vi "Acquire and Time.vi"(7 "samples per block":i64=-1, 8 "error in (no error)":errorcluster, 11 "RFSA Reference In":refnum<k15>) -> (0 "error out":errorcluster, 1 "bytes":i32, 2 "data":waveform(cdb), 3 "RFSA Reference Out":refnum<k15>, 5 "DAQ B/sec":dbl caption="ACQUISITION RATE")   [LabVIEW 2021]
uses:
  <instrlib>/niRFSA/niRFSA.llb/niRFSA Fetch IQ (Complex WDT 1Rec 1Chan).vi
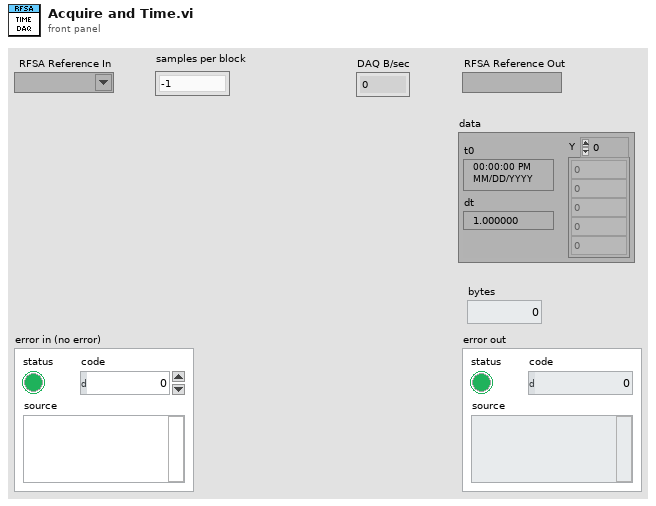
[diagram p1: front panel]
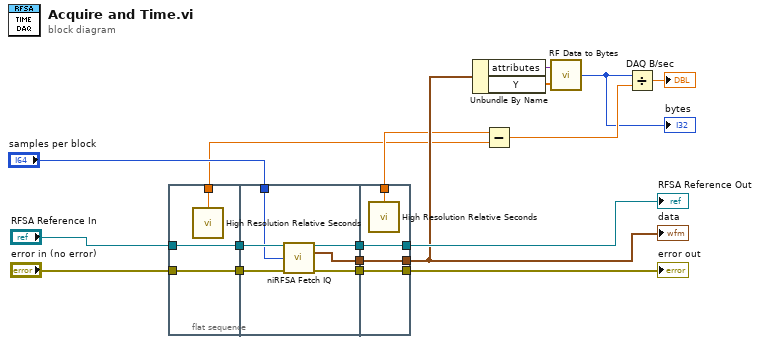
[diagram p0: block diagram]
diagram:
  n1 = flat-sequence {
    tunnel: [w19] -> w3
    tunnel: [w21] -> w18
    tunnel: "error in (no error)" -> [w21]
    tunnel: "RFSA Reference In" -> [w20]
    tunnel: [w20] -> w17
    tunnel: w18 -> [w27]
    tunnel: [w26] -> w16
    tunnel: [w25] -> w15
    tunnel: [w24] -> w14
    tunnel: w17 -> [w23]
    tunnel: "samples per block" -> [w22]
    tunnel: [w28] -> w4
    tunnel: w16 -> [w31]
    tunnel: [w31] -> w11
    tunnel: [w30] -> w5
    tunnel: w15 -> [w30]
    tunnel: w14 -> [w29]
    tunnel: [w29] -> w12
    frame #0 {
      n2 = call <vilib>:"High Resolution Relative Seconds.vi"() -> ("relative seconds"=w19:dbl)
    }
    frame #1 {
      n3 = call-poly <instrlib>:"niRFSA Fetch IQ.vi"("instrument handle"=w23, "samples to read (-1)"=w22, "error in"=w27) -> ("instrument handle out"=w24:refnum<k15>, "data"=w25:waveform(cdb), "error out"=w26:errorcluster)  [unwired: 10 in]
    }
    frame #2 {
      n4 = call <vilib>:"High Resolution Relative Seconds.vi"() -> ("relative seconds"=w28:dbl)
    }
  }
  n5 = Unbundle By Name(w5) -> ("attributes"=w7:variant, "Y"=w8:cdb[])
  n6 = Subtract(x=w4, y=w3) -> (x-y=w2:dbl)
  n7 = call "RF Data to Bytes.vi"("Y"=w8, "attributes"=w7) -> ("Bytes"=w1:i32)
  "bytes" <- w1
  n8 = Divide(x=w1, y=w2) -> (x/y=→"DAQ B/sec":dbl)
  "RFSA Reference Out" <- w12
  "data" <- w5
  "error out" <- w11
